vi "Subvi Event Log.vi"(0 "CustomMessage":string, 1 "EventNum":u32) -> ()   [LabVIEW 2012]
uses:
  ProSCI Global.vi
panel:
  # "Picks messages from a list\nbased on number. If num=0\ndisplays the custom message"
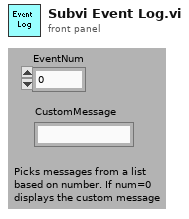
[diagram p1: front panel]
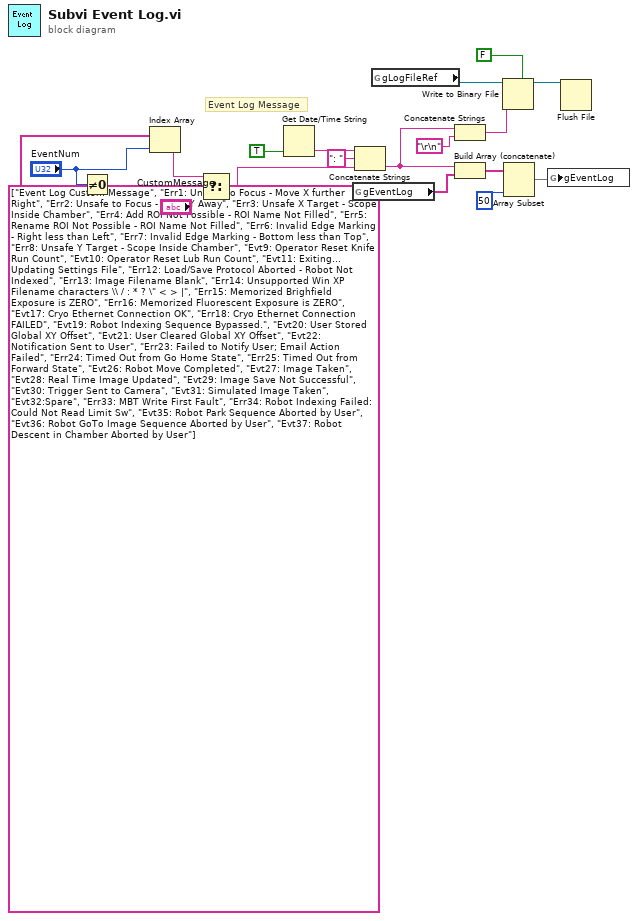
[diagram p0: block diagram]
diagram:
  # "Event Log Message"
  n1 = Not Equal To 0?(x="EventNum") -> (x != 0?=w6:bool)
  n2 = Index Array(array=string[] ["Event Log Custom Message", "Err1: Unsafe to Focus - Move X further Right", "Err2: Unsafe to Focus - Move Y Away", "Err3: Unsafe X Target - Scope Inside Chamber", "Err4: Add ROI Not Possible - ROI Name Not Filled", "Err5: Rename ROI Not Possible - ROI Name Not Filled", "Err6: Invalid Edge Marking - Right less than Left", "Err7: Invalid Edge Marking - Bottom less than Top", "Err8: Unsafe Y Target - Scope Inside Chamber", "Evt9: Operator Reset Knife Run Count", "Evt10: Operator Reset Lub Run Count", "Evt11: Exiting...Updating Settings File", "Err12: Load/Save Protocol Aborted - Robot Not Indexed", "Err13: Image Filename Blank", "Err14: Unsupported Win XP Filename characters \\ / : * ? \" < > |", "Err15: Memorized Brighfield Exposure is ZERO", "Err16: Memorized Fluorescent Exposure is ZERO", "Evt17: Cryo Ethernet Connection OK", "Err18: Cryo Ethernet Connection FAILED", "Evt19: Robot Indexing Sequence Bypassed.", "Evt20: User Stored Global XY Offset", "Evt21: User Cleared Global XY Offset", "Evt22: Notification Sent to User", "Err23: Failed to Notify User; Email Action Failed", "Err24: Timed Out from Go Home State", "Err25: Timed Out from Forward State", "Evt26: Robot Move Completed", "Evt27: Image Taken", "Evt28: Real Time Image Updated", "Evt29: Image Save Not Successful", "Evt30: Trigger Sent to Camera", "Evt31: Simulated Image Taken", "Evt32:Spare", "Err33: MBT Write First Fault", "Err34: Robot Indexing Failed: Could Not Read Limit Sw", "Evt35: Robot Park Sequence Aborted by User", "Evt36: Robot GoTo Image Sequence Aborted by User", "Evt37: Robot Descent in Chamber Aborted by User"], index="EventNum") -> (element=w5:string)
  n3 = Select(t=w5, s=w6, f="CustomMessage") -> (s? t:f=w3:string)
  n4 = Get Date/Time String(want seconds? (F)=TRUE) -> (time string=w17:string)  [unwired: 3 out]
  n5 = global read "ProSCI Global.vi" "gEventLog"() -> (w13:string[])
  n6 = Concatenate Strings(w17, ": " ("string"), w3) -> (w10:string)
  n7 = global read "ProSCI Global.vi" "gLogFileRef"() -> (w11:refnum<file>)
  n8 = Concatenate Strings(w10, "\r\n") -> (w9:string)
  n9 = Build Array (concatenate)(w10, w13) -> (w15:string[])
  n10 = Write to Binary File ("Write File")(file (use dialog)=w11, data=w9, 5:FALSE ("prepend array or string size? (T)")) -> (refnum out=w2:refnum<file>)  [unwired: 1 in, 4 out]
  n11 = Array Subset(array=w15, length=50) -> (w12:string[])  [unwired: 1 in]
  n12 = global write "ProSCI Global.vi" "gEventLog"(w12) -> ()
  n13 = Flush File(refnum=w2) -> ()  [unwired: 1 in, 2 out]
